vi "SetAccel.vi"(8 "error in (no error)":errorcluster, 11 "DelayLineLS4 in":refnum<class "DLLS4.lvclass">) -> (0 "error out":errorcluster, 3 "DelayLineLS4 out":refnum<class "DLLS4.lvclass">)   [LabVIEW 2019, in "DLLS4.lvclass"]
uses:
  DLLS4.lvclass
  C:/Users/elysium/Documents/dev/TRANCON/Classes/Delay Line/DelayLine.lvclass
  C:/Users/elysium/Documents/dev/TRANCON/Classes/GeneralFunctionality/GeneralFunctionality.lvclass
  LS4_parameters.ctl
  GeneralFunctionality/GeneralFunctionality.lvclass/GeneralFunctionality.ctl
  DelayLine.lvclass/DelayLine.ctl
  <vilib>/Utility/error.llb/DialogType.ctl
  Config/Config.lvclass
  <vilib>/ErrorRing/Error Ring.xnode
  DelayLine.lvclass
  GeneralFunctionality/GeneralFunctionality.lvclass
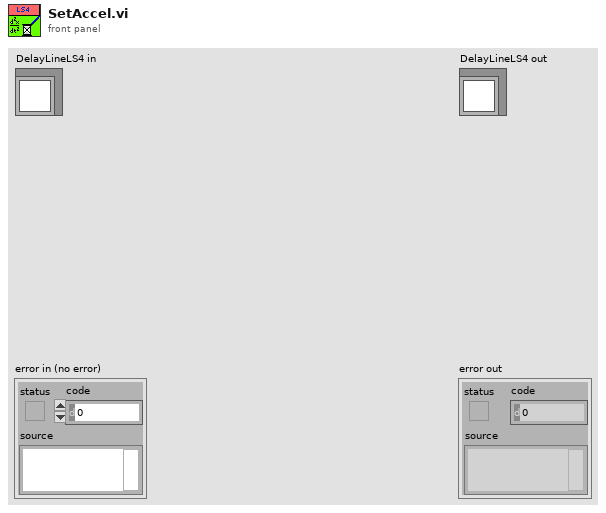
[diagram p1: front panel]
types:
  T1 = typedef "DelayLine.lvclass/LS4_parameters.ctl" = string
  T2 = typedef "DialogType.ctl" = u16
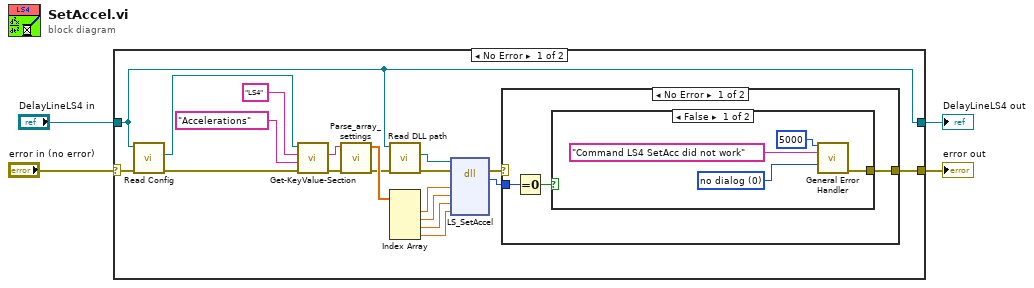
[diagram p0: block diagram]
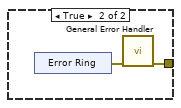
[diagram p2: hidden frame]
diagram:
  n1 = case shown="No Error" "error in (no error)" {
    selector: "error in (no error)" -> [w13 w36]
    tunnel: [w15 w36] -> w3
    tunnel: [w14 w35] -> w1
    tunnel: "DelayLineLS4 in" -> [w14 w35]
    frame No Error {
      n2 = call "Read Config.vi"("error in (no error)"=w13, "GeneralFunctionality en entrée"=w14) -> ("error out"=w7:errorcluster, "Config.lvclass"=w6:refnum<class "Config.lvclass">)  [unwired: 7 in, 1 out]
      n3 = call-dynamic "Get-KeyValue-Section.vi"("error in (no error)"=w7, "Key"=T1 "Accelerations" ("Section"), "Section"="LS4", "Config in"=w6) -> ("error out"=w5:errorcluster, "Value"=w10:string)  [unwired: 5 in, 1 out]
      n4 = call "Parse_array_settings.vi"("error in (no error)"=w5, "Value"=w10) -> ("error out"=w8:errorcluster, "Array"=w9:sgl[])  [unwired: 8 in]
      n5 = call "Read DLL path.vi"("error in (no error)"=w8, "DelayLine in"=w14) -> ("error out"=w17:errorcluster, "DLL path"=w16:path)  [unwired: 7 in, 1 out]
      n6 = Index Array(array=w9) -> (element #1=w20:sgl, element #2=w21:sgl, element #3=w22:sgl, element #4=w23:sgl)  [unwired: 4 in]
      n7 = dll-call lib="S:/TRANCON/DLL/LStep4.dll" fn="LS_SetAccel"(path in=w16, error in=w17, "X"=w20, "Y"=w21, "Z"=w22, "A"=w23) -> (error out=w19:errorcluster, "return type"=w18:i32)  [unwired: 5 in, 1 out]
      n8 = case shown="No Error" w19 {
        selector: w19 -> [_ w34]
        tunnel: w18 -> [w26 _]
        tunnel: [w24 w34] -> w15
        frame No Error {
          n9 = Equal To 0?(x=w26) -> (x = 0?=w25:bool)
          n10 = case shown="False" w25 {
            tunnel: [w28 w31] -> w24
            frame False {
              w27 = T2 0 items=["no dialog", "OK message", "continue or stop message", "OK message + warnings", "continue/stop + warnings"] ("type of dialog (OK msg:1)")
              n11 = call <vilib>:"General Error Handler.vi"("[error code] (0)"=5000 ("code"), "[error source] (\" \")"="Command LS4 SetAcc did not work" ("String to Prepend to source (\"\")"), "type of dialog (OK msg:1)"=w27) -> ("error out"=w28:errorcluster)  [unwired: 8 in, 4 out]
            }
            frame True {
              n12 = xnode "Error Ring"() -> ("error out"=w32:errorcluster)
              n13 = call <vilib>:"General Error Handler.vi"("error in (no error)"=w32) -> ("error out"=w31:errorcluster)  [unwired: 10 in, 4 out]
            }
          }
        }
        frame Error {
        }
      }
    }
    frame Error {
    }
  }
  "error out" <- w3
  "DelayLineLS4 out" <- w1
